vi "Auto Elevator Logic.vi"(6 "Presets":T1, 8 "Has Trashcan?":bool, 9 "Tote Count":i32, 10 "Elevator Sensors In":T3, 11 "Command":T5) -> (0 "Trashcan Delta":i32, 1 "Tote Count Delta":i32, 2 "Elevator Actuators Out":T2, 3 "State":T4)   [LabVIEW 2014]
uses:
  Elevator Command.ctl
  Common Code/Elevator State.ctl
  Elevator Actuators.ctl
  Common Code/Change Detect Int.vi
panel:
  in  "# Totes Loading":i32
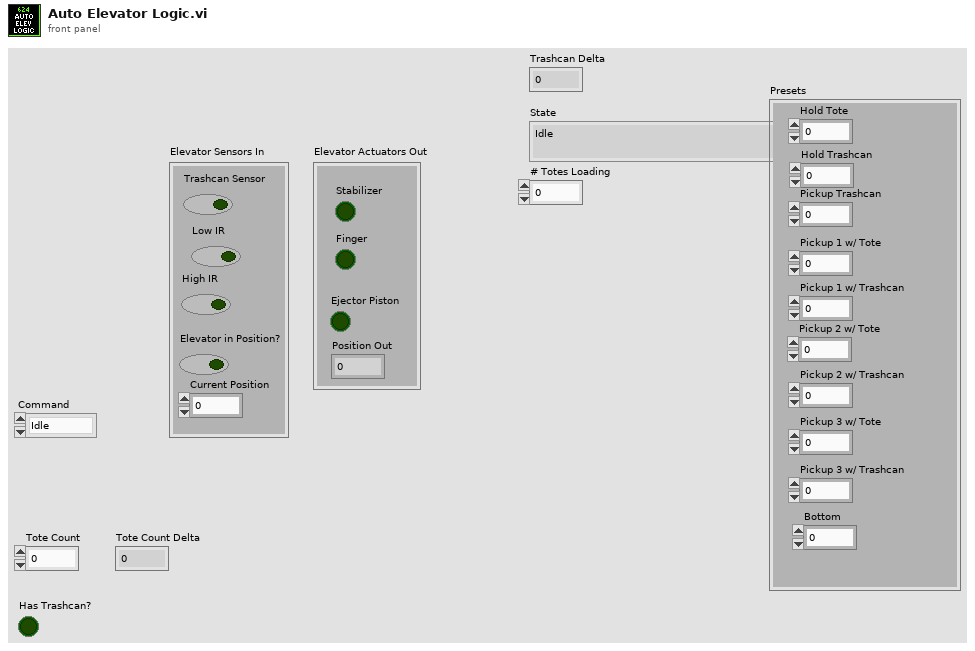
[diagram p1: front panel]
types:
  T1 = cluster{"Hold Tote":dbl, "Hold Trashcan":dbl, "Pickup 2 w/ Tote":dbl, "Pickup 2 w/ Trashcan":dbl, "Pickup 3 w/ Tote":dbl, "Pickup 3 w/ Trashcan":dbl, "Bottom":dbl, "Pickup 1 w/ Tote":dbl, "Pickup Trashcan":dbl, "Pickup 1 w/ Trashcan":dbl}
  T2 = typedef "Elevator Actuators.ctl" = cluster{"Ejector Piston":bool, "Finger":bool, "Stabilizer":bool, "Position Out":dbl}
  T3 = cluster{"Trashcan Sensor":bool, "Low IR":bool, "High IR":bool, "Elevator in Position?":bool, "Current Position":dbl}
  T4 = typedef "Elevator State.ctl" = enum16{"Idle", "Goto Load Position", "Wait for Load", "Load Drop", "Load Lift", "Drop Stack"}
  T5 = typedef "Elevator Command.ctl" = enum16{"Idle", "Load 1", "Load 2", "Load 3", "Drop Stack", "Eject Stack", "Load Trashcan"}
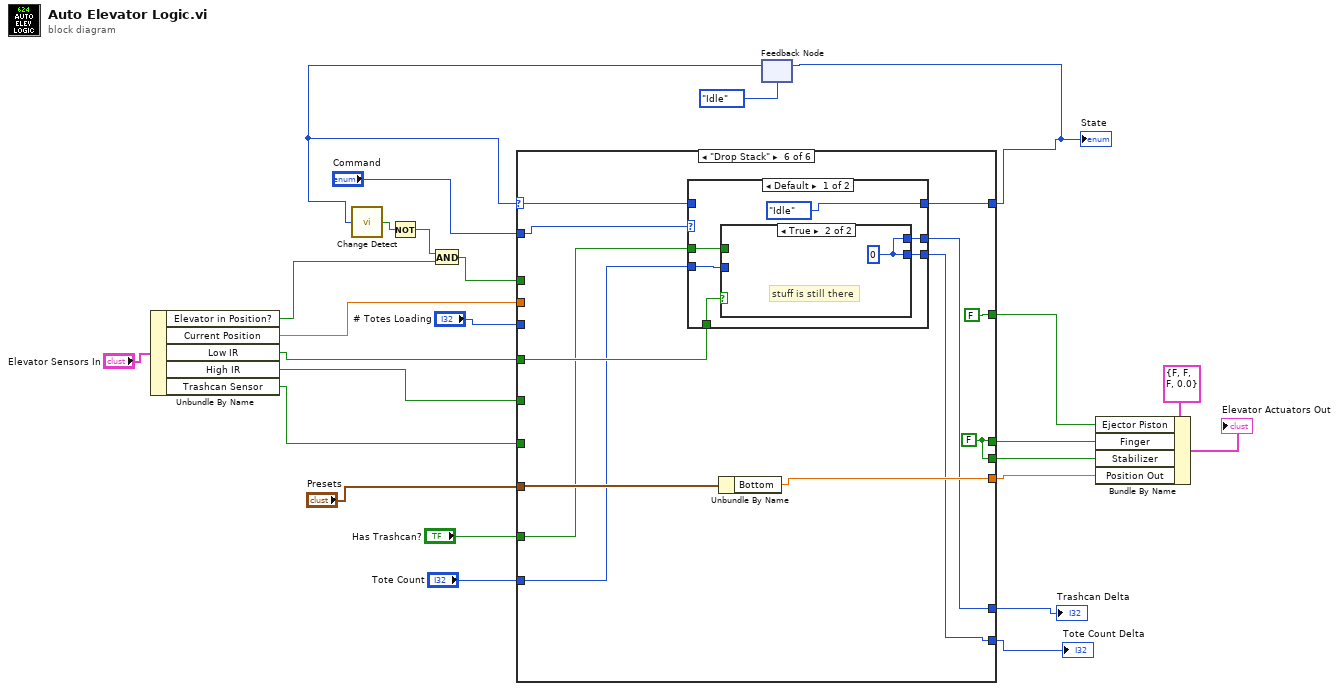
[diagram p0: block diagram]
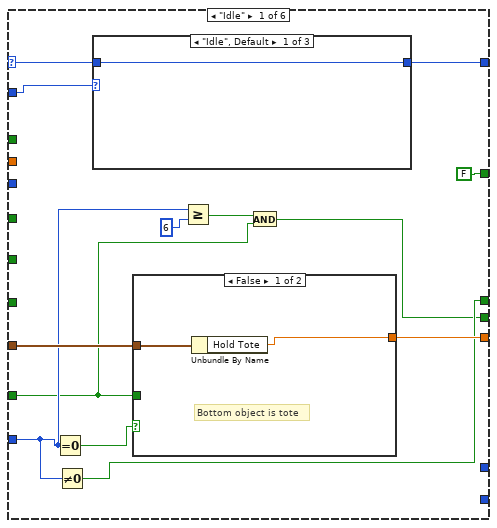
[diagram p2: hidden frame]
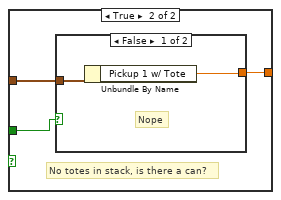
[diagram p3: hidden frame]
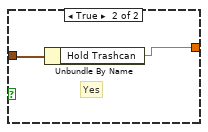
[diagram p4: hidden frame]
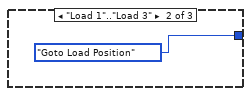
[diagram p5: hidden frame]
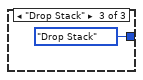
[diagram p6: hidden frame]
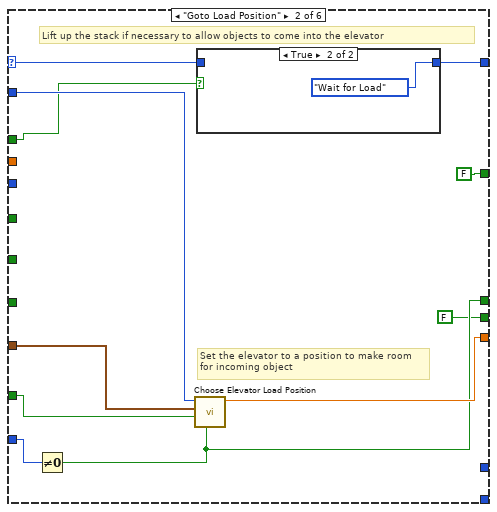
[diagram p7: hidden frame]
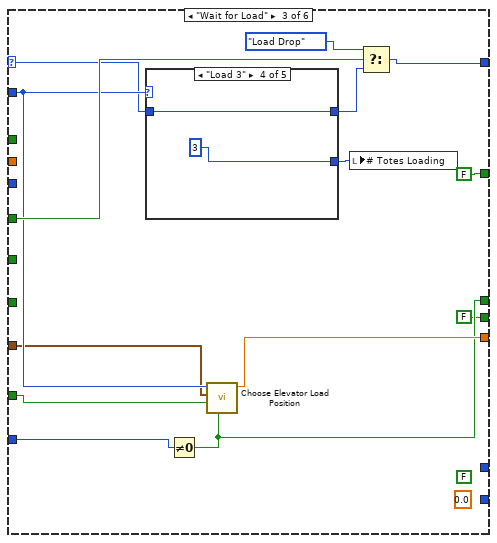
[diagram p9: hidden frame]
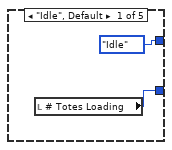
[diagram p10: hidden frame]
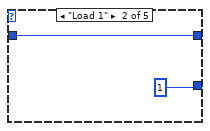
[diagram p11: hidden frame]
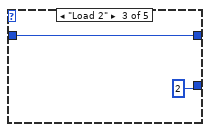
[diagram p12: hidden frame]
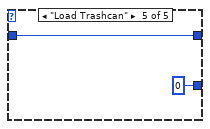
[diagram p13: hidden frame]
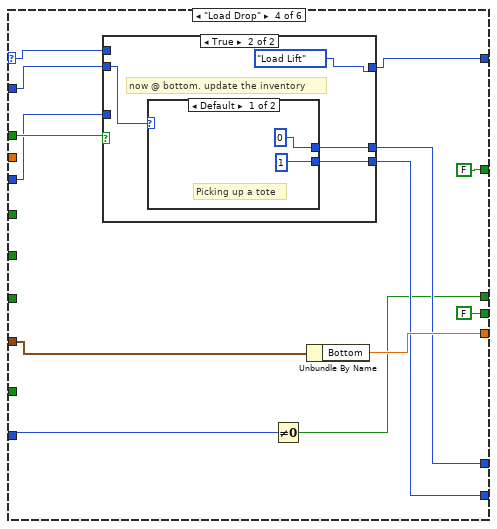
[diagram p14: hidden frame]
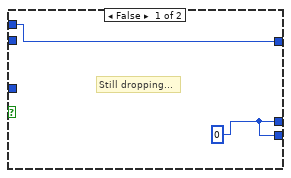
[diagram p15: hidden frame]
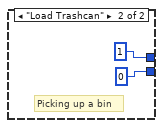
[diagram p16: hidden frame]
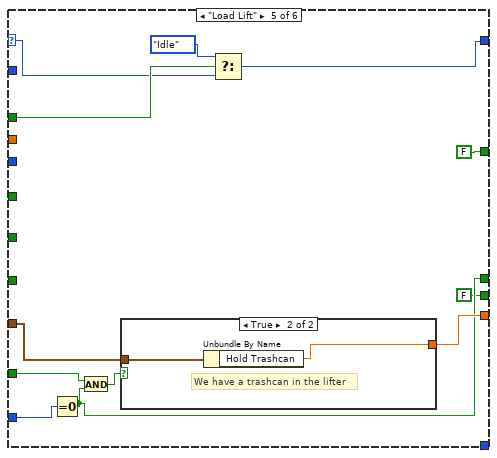
[diagram p17: hidden frame]
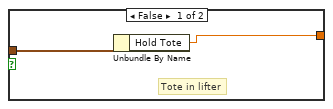
[diagram p18: hidden frame]
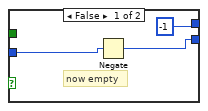
[diagram p19: hidden frame]
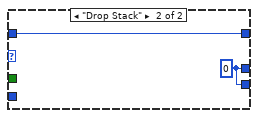
[diagram p20: hidden frame]
diagram:
  n1 = Unbundle By Name("Elevator Sensors In") -> ("Elevator in Position?"=w17:bool, "Current Position"=w14:dbl, "Low IR"=w16:bool, "High IR"=w15:bool, "Trashcan Sensor"=w13:bool)
  n2 = feedback #1(Elevator_State."Idle" ("Enum")) -> (w19:T4)
  n3 = call-poly "Change Detect.vi"("In"=w19) -> ("Changed?"=w22:bool)
  n4 = Not(x=w22) -> (.not. x?=w21:bool)
  n5 = And(x=w21, y=w17) -> (x .and. y?=w23:bool)
  n6 = case shown="\"Drop Stack\"" w19 {
    selector: w19 -> [w36 w58 w71 w91 w117 w134]
    tunnel: [w35 w57 w73 w92 w116 w133] -> w3
    tunnel: [FALSE ("Ejector Piston") FALSE ("Ejector Piston") FALSE ("Ejector Piston") FALSE ("Ejector Piston") FALSE ("Ejector Piston") FALSE ("Ejector Piston")] -> w6
    tunnel: "Presets" -> [w34 w55 w66 w96 w121 w137]
    tunnel: [w33 w60 w77 w99 w120 w136] -> w7
    tunnel: w14 -> [_ _ _ _ _ _]
    tunnel: w16 -> [_ _ w75 _ _ w132]
    tunnel: w15 -> [_ _ _ _ _ _]
    tunnel: "Command" -> [w37 w61 w72 w93 _ w135]
    tunnel: w23 -> [_ w56 _ w98 w118 _]
    tunnel: "# Totes Loading" -> [_ _ _ w97 _ _]
    tunnel: w13 -> [_ _ _ _ _ _]
    tunnel: "Has Trashcan?" -> [w27 w54 w67 _ w114 w131]
    tunnel: "Tote Count" -> [w30 w53 w68 w90 w113 w130]
    tunnel: [_ _ _ w94 _ w129] -> w5
    tunnel: [_ _ _ w95 _ w128] -> w4
    tunnel: [w31 w52 w65 w89 w112 w127] -> w2
    tunnel: [w26 FALSE FALSE FALSE FALSE w127] -> w1
    frame "Idle" {
      n7 = Equal To 0?(x=w30) -> (x = 0?=w32:bool)
      n8 = Not Equal To 0?(x=w30) -> (x != 0?=w31:bool)
      n9 = case shown="\"Idle\", Default" w37 {
        tunnel: w36 -> [w48 _ _]
        tunnel: [w48 Elevator_State."Goto Load Position" ("Enum") Elevator_State."Drop Stack" ("Enum")] -> w35
        frame "Idle", Default {
        }
        frame "Load 1".."Load 3" {
        }
        frame "Drop Stack" {
        }
      }
      n10 = case shown="False" w32 {
        tunnel: w34 -> [w40 w43]
        tunnel: [w39 w42] -> w33
        tunnel: w27 -> [_ w41]
        frame False {
          # "Bottom object is tote"
          n11 = Unbundle By Name(w40) -> ("Hold Tote"=w39:dbl)
        }
        frame True {
          # "No totes in stack, is there a can?"
          n12 = case shown="False" w41 {
            tunnel: w43 -> [w45 w47]
            tunnel: [w44 w46] -> w42
            frame False {
              # "Nope"
              n13 = Unbundle By Name(w45) -> ("Pickup 1 w/ Tote"=w44:dbl)
            }
            frame True {
              # "Yes"
              n14 = Unbundle By Name(w47) -> ("Hold Trashcan"=w46:dbl)
            }
          }
        }
      }
      n15 = Greater Or Equal?(x=w30, y=6) -> (x >= y?=w28:bool)
      n16 = And(x=w28, y=w27) -> (x .and. y?=w26:bool)
    }
    frame "Goto Load Position" {
      # "Set the elevator to a position to make room\nfor incoming object"
      # "Lift up the stack if necessary to allow objects to come into the elevator"
      n17 = Not Equal To 0?(x=w53) -> (x != 0?=w52:bool)
      n18 = call "Choose Elevator Load Position.vi"("Have Totes?"=w52, "Have Trashcan?"=w54, "Presets"=w55, "Command"=w61) -> ("Elevator Position"=w60:dbl)  [unwired: 7 in]
      n19 = case shown="True" w56 {
        tunnel: w58 -> [w62 _]
        tunnel: [w62 Elevator_State."Wait for Load" ("Enum")] -> w57
        frame False {
          # "Wait on elevator..."
        }
        frame True {
        }
      }
    }
    frame "Wait for Load" {
      (unwired) 0.0
      (unwired) FALSE
      n20 = case shown="\"Load 3\"" w72 {
        tunnel: w71 -> [_ w81 w83 w85 w86]
        tunnel: [Elevator_State."Idle" ("Enum") w81 w83 w85 w86] -> w70
        tunnel: [w79 1 2 3 0 ("# Totes Loading")] -> w69
        frame "Idle", Default {
          n21 = local read "# Totes Loading"() -> (w79:i32)
        }
        frame "Load 1" {
        }
        frame "Load 2" {
        }
        frame "Load 3" {
        }
        frame "Load Trashcan" {
        }
      }
      n22 = Not Equal To 0?(x=w68) -> (x != 0?=w65:bool)
      n23 = call "Choose Elevator Load Position.vi"("Have Totes?"=w65, "Have Trashcan?"=w67, "Presets"=w66, "Command"=w72) -> ("Elevator Position"=w77:dbl)  [unwired: 7 in]
      n24 = local write "# Totes Loading"(w69) -> ()
      n25 = Select(t=Elevator_State."Load Drop" ("Enum"), s=w75, f=w70) -> (s? t:f=w73:T4)
    }
    frame "Load Drop" {
      n26 = case shown="True" w98 {
        tunnel: w93 -> [_ w106]
        tunnel: w97 -> [_ _]
        tunnel: [w102 w105] -> w95
        tunnel: [w102 w104] -> w94
        tunnel: [w101 Elevator_State."Load Lift" ("Enum")] -> w92
        tunnel: w91 -> [w101 _]
        frame False {
          w102 = 0
          # "Still dropping..."
        }
        frame True {
          # "now @ bottom. update the inventory"
          n27 = case shown="Default" w106 {
            tunnel: [0 1] -> w105
            tunnel: [1 0] -> w104
            frame Default {
              # "Picking up a tote"
            }
            frame "Load Trashcan" {
              # "Picking up a bin"
            }
          }
        }
      }
      n28 = Not Equal To 0?(x=w90) -> (x != 0?=w89:bool)
      n29 = Unbundle By Name(w96) -> ("Bottom"=w99:dbl)
    }
    frame "Load Lift" {
      n30 = Equal To 0?(x=w113) -> (x = 0?=w112:bool)
      n31 = And(x=w114, y=w112) -> (x .and. y?=w119:bool)
      n32 = case shown="True" w119 {
        tunnel: w121 -> [w124 w126]
        tunnel: [w123 w125] -> w120
        frame False {
          # "Tote in lifter"
          n33 = Unbundle By Name(w124) -> ("Hold Tote"=w123:dbl)
        }
        frame True {
          # "We have a trashcan in the lifter"
          n34 = Unbundle By Name(w126) -> ("Hold Trashcan"=w125:dbl)
        }
      }
      n35 = Select(t=Elevator_State."Idle", s=w118, f=w117) -> (s? t:f=w116:T4)
    }
    frame "Drop Stack" {
      w127 = FALSE
      n36 = case shown="Default" w135 {
        tunnel: w134 -> [_ w150]
        tunnel: [Elevator_State."Idle" ("Enum") w150] -> w133
        tunnel: [w142 w149] -> w129
        tunnel: w132 -> [w143 _]
        tunnel: w131 -> [w141 _]
        tunnel: w130 -> [w140 _]
        tunnel: [w139 w149] -> w128
        frame Default {
          n37 = case shown="True" w143 {
            tunnel: [w145 w148] -> w142
            tunnel: w141 -> [_ _]
            tunnel: w140 -> [w146 _]
            tunnel: [-1 w148] -> w139
            frame False {
              # "now empty"
              n38 = Negate(x=w146) -> (-x=w145:i32)
            }
            frame True {
              w148 = 0
              # "stuff is still there"
            }
          }
        }
        frame "Drop Stack" {
          w149 = 0
        }
      }
      n39 = Unbundle By Name(w137) -> ("Bottom"=w136:dbl)
    }
  }
  "Tote Count Delta" <- w5
  "State" <- w3
  "Trashcan Delta" <- w4
  n40 = feedback-in #1(w3) -> ()
  n41 = Bundle By Name(cluster=T2 {"Ejector Piston"=FALSE, "Finger"=FALSE, "Stabilizer"=FALSE, "Position Out"=0.0} ("Elevator Actuators Out"), "Ejector Piston"=w6, "Finger"=w2, "Stabilizer"=w1, "Position Out"=w7) -> (→"Elevator Actuators Out":T2)
